vi "Check Module Config.vi"(5 "EtherCAT?":bool, 7 "R/W Case":T4, 8 "error in (no error)":errorcluster, 11 "Module Config Data in":T1 {"Config Block Data Refs"."Data Reference" format="%.0x"}) -> (0 "error out":errorcluster, 3 "Module Config Data out":T1 {"Config Block Data Refs"."Data Reference" format="%.0x"})   [LabVIEW 2016, in "Scan Engine Custom Device.lvlib"]
uses:
  Scan Engine Custom Device.lvlib
  Type Defs/RW Case.ctl
  Type Defs/Module Config Data.ctl
  <vilib>/NI Veristand/Custom Device API/Block Data Reference.ctl
  <vilib>/NI Veristand/Custom Device API/Data Reference.ctl
  <vilib>/NI Veristand/Custom Device API/Global Data Refs.vi
  <vilib>/NI Veristand/Custom Device API/Custom Device API.lvlib
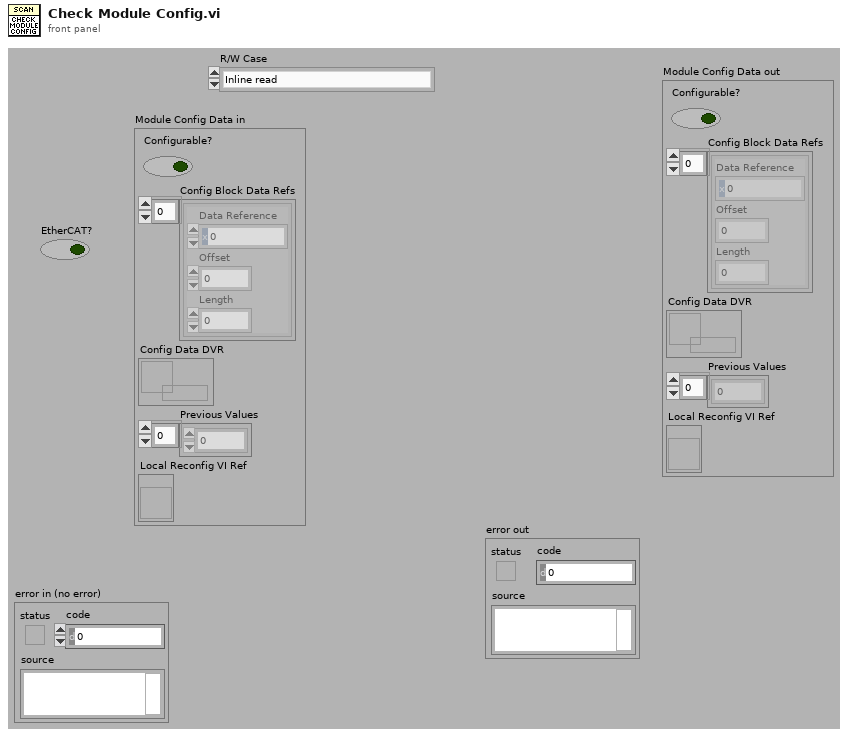
[diagram p1: front panel]
types:
  T1 = typedef "Scan Engine Custom Device.lvlib/Module Config Data.ctl" = cluster{"Configurable?":bool, "Config Block Data Refs":T2[], "Config Data DVR":refnum<data-value>, "Previous Values":dbl[], "Local Reconfig VI Ref":refnum<vi>}
  T2 = typedef "Custom Device API.lvlib/Block Data Reference.ctl" = cluster{"Data Reference":T3, "Offset":u64, "Length":u64}
  T3 = typedef "Custom Device API.lvlib/Data Reference.ctl" = i32
  T4 = typedef "Scan Engine Custom Device.lvlib/RW Case.ctl" = enum16{"Inline read", "Inline write", "Async - Inline loop read", "Async - Inline loop write", "Async loop (read/write)"}
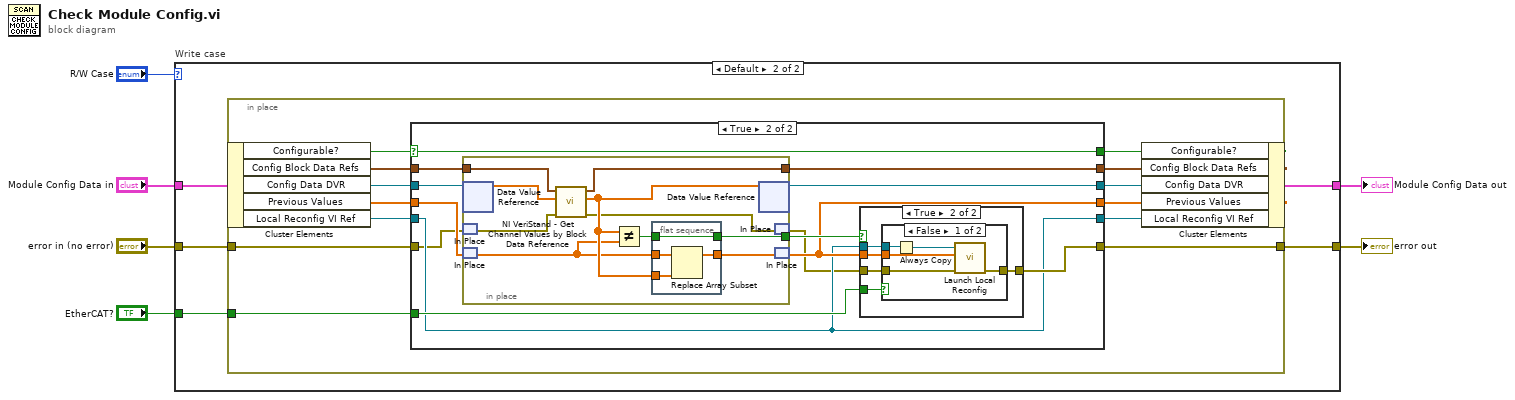
[diagram p0: block diagram]
diagram:
  n1 = case "Write case" shown="Default" "R/W Case" {
    tunnel: "Module Config Data in" -> [w7 w13]
    tunnel: "error in (no error)" -> [w8 w12]
    tunnel: [w8 w11] -> w6
    tunnel: [w7 w10] -> w2
    tunnel: "EtherCAT?" -> [_ w9]
    frame "Async loop (read/write)" {
    }
    frame Default {
      n2 = in-place {
        in-place-border: w12 -> [w26]
        in-place-border: [w24] -> w11
        in-place-border: w9 -> [w16]
        n3 = in-place-cluster #1(w13) -> ("Configurable?"=w23:bool, "Config Block Data Refs"=w25:T2[], "Config Data DVR"=w22:refnum<data-value>, "Previous Values"=w18:dbl[], "Local Reconfig VI Ref"=w14:refnum<vi>)
        n4 = case shown="True" w23 {
          selector: w23 -> [w29 w41]
          tunnel: w26 -> [w32 w34]
          tunnel: w25 -> [w31 w45]
          tunnel: [w32 w37] -> w24
          tunnel: w22 -> [w30 w44]
          tunnel: [w31 w43] -> w21
          tunnel: [w30 w42] -> w20
          tunnel: [w29 w41] -> w19
          tunnel: w18 -> [w28 w38]
          tunnel: [w28 w36] -> w17
          tunnel: w16 -> [_ w40]
          tunnel: [w27 w35] -> w15
          tunnel: w14 -> [w27 w35]
          frame False {
          }
          frame True {
            n5 = in-place {
              in-place-border: w45 -> [w67]
              in-place-border: [w66] -> w43
              in-place-border: [w63] -> w39
              n6 = in-place-dvr #2(w44) -> (w65:dbl[])  [unwired: 1 out]
              n7 = in-place-match #3(w34) -> (w59:errorcluster)
              n8 = in-place-match #4(w38) -> (w61:dbl[])
              n9 = call <vilib>:"NI VeriStand - Get Channel Values by Block Data Reference.vi"("error in (no error)"=w59, "Values Array in"=w65, "Block Data Ref"=w67) -> ("error out"=w58:errorcluster, "Values Array out"=w62:dbl[], "Block Data Ref dup"=w66:T2[])  [unwired: 6 in]
              n10 = Not Equal?(x=w62, y=w61) -> (x != y?=w64:bool)
              n11 = flat-sequence {
                tunnel: w64 -> [w71]
                tunnel: [w71] -> w63
                tunnel: w61 -> [w70]
                tunnel: w62 -> [w69]
                tunnel: [w68] -> w60
                frame #0 {
                  n12 = Replace Array Subset(array=w70, new element=w69) -> (w68:dbl[])  [unwired: 1 in]
                }
              }
              n13 = in-place-dvr #2(w62) -> (w42:refnum<data-value>)  [unwired: 1 out]
              n14 = in-place-match #3(w58) -> (w33:errorcluster)
              n15 = in-place-match #4(w60) -> (w36:dbl[])
            }
            n16 = case shown="True" w39 {
              tunnel: w40 -> [_ w51]
              tunnel: w36 -> [_ w50]
              tunnel: w33 -> [w46 w49]
              tunnel: w35 -> [_ w48]
              tunnel: [w46 w47] -> w37
              frame False {
              }
              frame True {
                n17 = case shown="False" w51 {
                  tunnel: w50 -> [w53 _]
                  tunnel: w49 -> [w55 w57]
                  tunnel: w48 -> [w56 _]
                  tunnel: [w54 w57] -> w47
                  frame False {
                    n18 = Always Copy(1:w56) -> (0:w52:refnum<vi>)
                    n19 = call "Launch Local Reconfig.vi"("error in (no error)"=w55, "Config Channels"=w53, "Local Reconfig VI Ref"=w52) -> ("error out"=w54:errorcluster)  [unwired: 8 in]
                  }
                  frame True {
                  }
                }
              }
            }
          }
        }
        n20 = in-place-cluster #1("Configurable?"=w19, "Config Block Data Refs"=w21, "Config Data DVR"=w20, "Previous Values"=w17, "Local Reconfig VI Ref"=w15) -> (w10:T1)
      }
    }
  }
  "error out" <- w6
  "Module Config Data out" <- w2
